vi "TM update all.vi"(8 "error in (no error)":errorcluster, 11 "VISA Refnum in":refnum<visa-resource-name>) -> (0 "error out":errorcluster, 2 "LSC218 sensors":T1 {"Time stamp" format="%<%H:%M:%S%2u\n%Y/%m/%d>T"}, 3 "VISA Refnum out":refnum<visa-resource-name>)   [LabVIEW 2021, in "Temperature monitor.lvlib"]
doc: "Queries Temperature monitor (LSC218) for all values from sensors in cryostat."
uses:
  ctl/Cryostat temperature sensors.ctl
  Temperature monitor.lvlib
  <instrlib>/Lake Shore 218/Lake Shore Cryotronics 218.lvlib
  Magnet module.lvlib
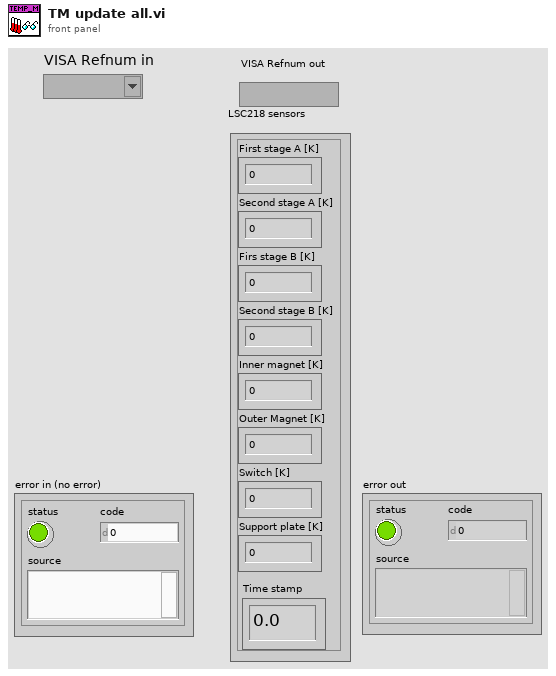
[diagram p1: front panel]
types:
  T1 = typedef "Magnet module.lvlib/Cryostat temperature sensors.ctl" = cluster{"First stage A [K]":dbl, "Second stage A [K]":dbl, "Firs stage B [K]":dbl, "Second stage B [K]":dbl, "Inner magnet [K]":dbl, "Outer Magnet [K]":dbl, "Switch [K]":dbl, "Support plate [K]":dbl, "Time stamp":dbl}
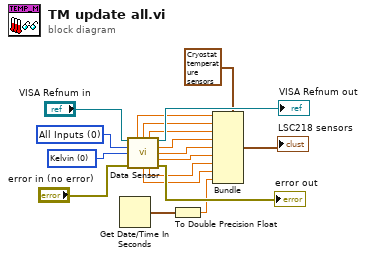
[diagram p0: block diagram]
diagram:
  w2 = u16 0 items=["Kelvin", "Celsius", "Sensor Units", "Linear Data"] ("Data Source (0:Kelvin)")
  w3 = u16 0 items=["All Inputs", "1", "2", "3", "4", "5", "6", "7", "8"] ("Input (0:All)")
  n1 = Get Date/Time In Seconds() -> (seconds since 1Jan1904=w4:timestamp)
  n2 = call <instrlib>:"Data Sensor.vi"("VISA resource name"="VISA Refnum in", "Input (0:All)"=w3, "Data Source (0:Kelvin)"=w2, "error in (no error)"="error in (no error)") -> ("Input 1"=w7:dbl, "Input 2"=w8:dbl, "Input 3"=w9:dbl, "VISA resource name out"=→"VISA Refnum out":refnum<visa-resource-name>, "Input 4"=w10:dbl, "Input 5"=w11:dbl, "Input 6"=w12:dbl, "Input 8"=w14:dbl, "Input 7"=w13:dbl, "error out"=→"error out":errorcluster)  [unwired: 2 in]
  n3 = To Double Precision Float(number=w4) -> (double precision float=w1:dbl)
  n4 = Bundle(cluster=T1 {"First stage A [K]"=0.0, "Second stage A [K]"=0.0, "Firs stage B [K]"=0.0, "Second stage B [K]"=0.0, "Inner magnet [K]"=0.0, "Outer Magnet [K]"=0.0, "Switch [K]"=0.0, "Support plate [K]"=0.0, "Time stamp"=0.0} ("LSC218 sensors"), "First stage A [K]"=w7, "Second stage A [K]"=w8, "Firs stage B [K]"=w9, "Second stage B [K]"=w10, "Inner magnet [K]"=w11, "Outer Magnet [K]"=w12, "Switch [K]"=w13, "Support plate [K]"=w14, "Time stamp"=w1) -> (→"LSC218 sensors":T1)
